vi "createRegisters.vi"() -> (4 "registers":T1={"PLLGains"="PLLGains", "PLLRange"="PLLRange", "PLL_reset"="PLL_reset", "PLL_locked"="PLL_locked", "freqBoundaries"="freqBoundaries", "expectedFreq"="expectedFreq", "lockDuration"="lockDuration", "dT"="dT", "detectedFreq"="detectedFreq", "adjustTheta"="adjustTheta", "HarmonicFilter"="HarmonicFilter", "HarmonicFilterEnable"="HarmonicFilterEnable"})   [LabVIEW 2017, in "ThreePhasePLL.lvlib"]
uses:
  ThreePhasePLL.lvlib
  registers.ctl
  <vilib>/rvi/eio/common/nirviEmuReportErrorAndStop.vi
  <vilib>/rvi/DataTransferAndStorage/Container/Common/niFpgaContainerSetEmuInfo.vi
  <vilib>/rvi/DataTransferAndStorage/Container/Common/niFpgaContainerGetUniqueNameForEmu.vi
  <vilib>/rvi/LocalResourceManager/LocalResourceManager.xnode
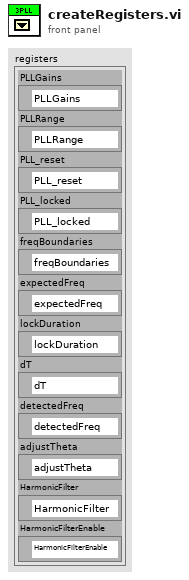
[diagram p1: front panel]
types:
  T1 = typedef "ThreePhasePLL.lvlib/registers.ctl" = cluster{"PLLGains":refnum<k21>, "PLLRange":refnum<k21>, "PLL_reset":refnum<k21>, "PLL_locked":refnum<k21>, "freqBoundaries":refnum<k21>, "expectedFreq":refnum<k21>, "lockDuration":refnum<k21>, "dT":refnum<k21>, "detectedFreq":refnum<k21>, "adjustTheta":refnum<k21>, "HarmonicFilter":refnum<k21>, "HarmonicFilterEnable":refnum<k21>}
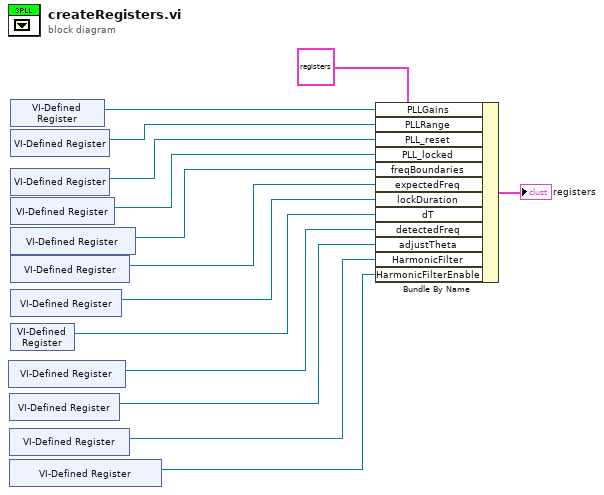
[diagram p0: block diagram]
diagram:
  n1 = xnode "VI-Defined Register"() -> ("Register Out"=w4:refnum<k21>)
  n2 = xnode "VI-Defined Register"() -> ("Register Out"=w3:refnum<k21>)
  n3 = xnode "VI-Defined Register"() -> ("Register Out"=w2:refnum<k21>)
  n4 = xnode "VI-Defined Register"() -> ("Register Out"=w1:refnum<k21>)
  n5 = xnode "VI-Defined Register"() -> ("Register Out"=w13:refnum<k21>)
  n6 = xnode "VI-Defined Register"() -> ("Register Out"=w12:refnum<k21>)
  n7 = xnode "VI-Defined Register"() -> ("Register Out"=w11:refnum<k21>)
  n8 = xnode "VI-Defined Register"() -> ("Register Out"=w10:refnum<k21>)
  n9 = xnode "VI-Defined Register"() -> ("Register Out"=w9:refnum<k21>)
  n10 = xnode "VI-Defined Register"() -> ("Register Out"=w8:refnum<k21>)
  n11 = xnode "VI-Defined Register"() -> ("Register Out"=w7:refnum<k21>)
  n12 = xnode "VI-Defined Register"() -> ("Register Out"=w6:refnum<k21>)
  n13 = Bundle By Name(cluster=T1 {"PLLGains"="", "PLLRange"="", "PLL_reset"="", "PLL_locked"="", "freqBoundaries"="", "expectedFreq"="", "lockDuration"="", "dT"="", "detectedFreq"="", "adjustTheta"="", "HarmonicFilter"="", "HarmonicFilterEnable"="HarmonicFilterEnable"} ("Cluster"), "PLLGains"=w13, "PLLRange"=w12, "PLL_reset"=w11, "PLL_locked"=w10, "freqBoundaries"=w9, "expectedFreq"=w8, "lockDuration"=w7, "dT"=w6, "detectedFreq"=w4, "adjustTheta"=w3, "HarmonicFilter"=w2, "HarmonicFilterEnable"=w1) -> (→"registers":T1)
